vi "Register Click Callback.vi"(8 "error in":errorcluster, 10 "onClick":refnum<user-event>, 11 "Custom Events in":refnum<class "Custom Events.lvclass">) -> (0 "error out":errorcluster, 2 "Event Callback Refnum":refnum<k27>, 3 "Custom Events out":refnum<class "Custom Events.lvclass">)   [LabVIEW 2023, in "SourceGrid.lvlib" / "Custom Events.lvclass"]
uses:
  Custom Events.lvclass
  Cells/Cell Context/Cell Context.lvclass
  Click Callback.vi
  D:/git/Sourcegrid-LabVIEW/dll/SourceGrid.dll
  dll/SourceGrid.dll
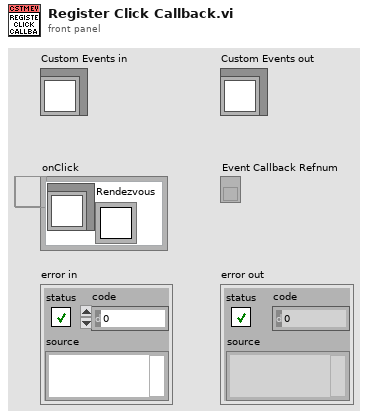
[diagram p1: front panel]
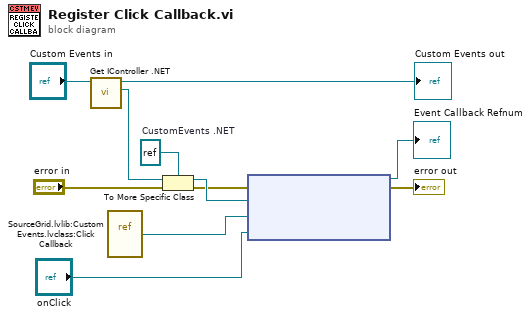
[diagram p0: block diagram]
diagram:
  w5 = refnum<k24> refnum  # CustomEvents .NET
  n1 = call-dynamic "Get IController .NET.vi"("Custom Events in"="Custom Events in") -> ("IController"=w4:refnum<k24>, "Custom Events out"=→"Custom Events out":refnum<class "Custom Events.lvclass">)  [unwired: 9 in]
  n2 = vi-ref "SourceGrid.lvlib:Custom Events.lvclass:Click Callback.vi"() -> (w6:refnum<vi>)
  n3 = To More Specific Class(target class=w5, reference=w4, error in="error in") -> (specific class reference=w3:refnum<k24>, error out=w1:errorcluster)
  n4 = node(w1, w3, w6, "onClick") -> (→"Event Callback Refnum":refnum<k27>, →"error out":errorcluster)  [unwired: 1 in]
